vi "QuitMode.vi"(1 "hide ftp and quit?":bool) -> (0 "mode":i32)   [LabVIEW 2022 SP3]
panel:
  in  "return":bool
  in  "quit":bool
  in  "ftpandquit":bool
  # "Warning! Unsaved data will be lost if Quit options are chosen. Unsaved data cannot be sent to RRI via FTP."
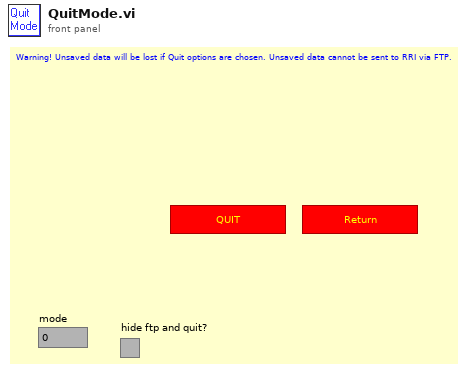
[diagram p1: front panel]
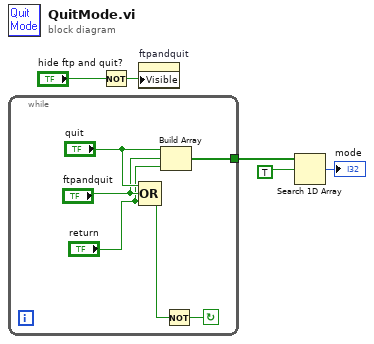
[diagram p0: block diagram]
diagram:
  n1 = while {
    tunnel: [w6] -> w3
    stop <- w10 continue-if-true
    n2 = Compound Arithmetic op=OR("quit", "ftpandquit", "return") -> (w11:bool)
    n3 = Build Array("quit", "ftpandquit", "return") -> (w6:bool[])
    n4 = Not(x=w11) -> (.not. x?=w10:bool)
  }
  n5 = Not(x="hide ftp and quit?") -> (.not. x?=w2:bool)
  n6 = property on="ftpandquit" class="Bool"("Visible"=w2) -> ()  [unwired: 2 in, 2 out]
  n7 = Search 1D Array(1D array=w3, element=TRUE) -> (index of element=→"mode":i32)  [unwired: 1 out]
